vi "Format Container ACL.vi"(11 "ACL":T1[](array[typedef])) -> (3 "ACL string":string)   [LabVIEW 2015, in "NI_Azure_Queue.lvlib"]
uses:
  NI_Azure_Queue.lvlib
  Signed Identifier.ctl
  Access Policy.ctl
  <vilib>/Utility/error.llb/whitespace.ctl
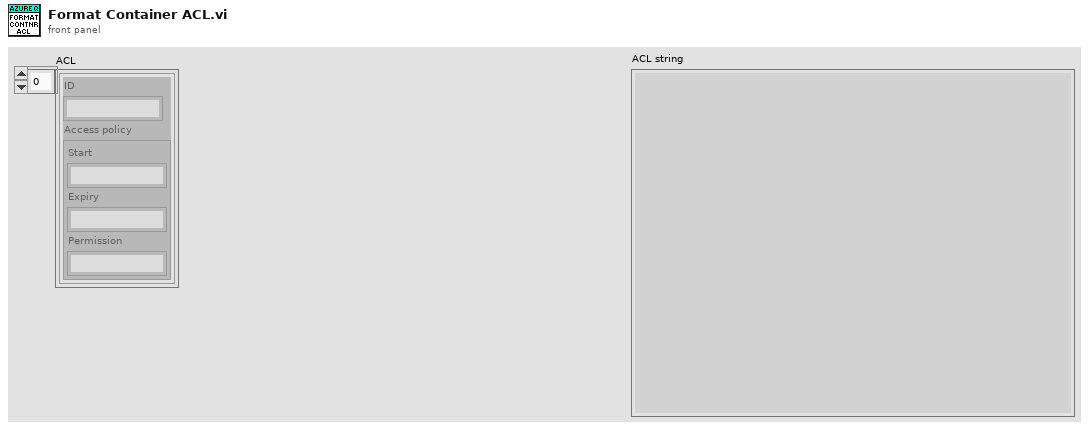
[diagram p1: front panel]
types:
  T1 = typedef "NI_Azure_Queue.lvlib/Signed Identifier.ctl" = cluster{"ID":string, "Access policy":T2}
  T2 = typedef "NI_Azure_Queue.lvlib/Access Policy.ctl" = cluster{"Start":string, "Expiry":string, "Permission":string}
  T3 = typedef "whitespace.ctl" = u16
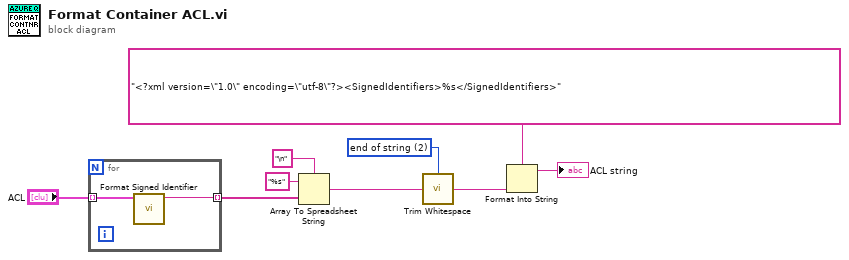
[diagram p0: block diagram]
diagram:
  w1 = T3 2 items=["both", "start of string", "end of string"] ("location (both)")
  n1 = for {
    tunnel: "ACL" -> [w11] mode=indexing
    tunnel: [w10] -> w6 mode=indexing
    n2 = call "Format Signed Identifier.vi"("Signed identifier"=w11) -> ("Signed identifier string"=w10:string)  [unwired: 10 in]
  }
  n3 = Array To Spreadsheet String(delimiter (Tab)="\n", array=w6, 3:"%s" ("format string")) -> (spreadsheet string=w3:string)
  n4 = call <vilib>:"Trim Whitespace.vi"("string"=w3, "location (both)"=w1) -> ("trimmed string"=w2:string)
  n5 = Format Into String(format string="<?xml version=\"1.0\" encoding=\"utf-8\"?><SignedIdentifiers>%s</SignedIdentifiers>", w2) -> (resulting string=→"ACL string":string)  [unwired: 2 in, 1 out]
